vi "Available_Machines.vi"(1 "Row Number":i32) -> (0 "Machine Names":string[](array[string]))   [LabVIEW 2010]
uses:
  ADAM Controls/Channel_names.ctl
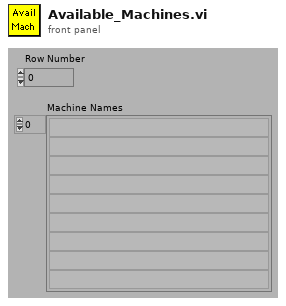
[diagram p1: front panel]
types:
  T1 = typedef "Channel_names.ctl" = enum16{"Active Only", "Active + Off", "All Channels"}
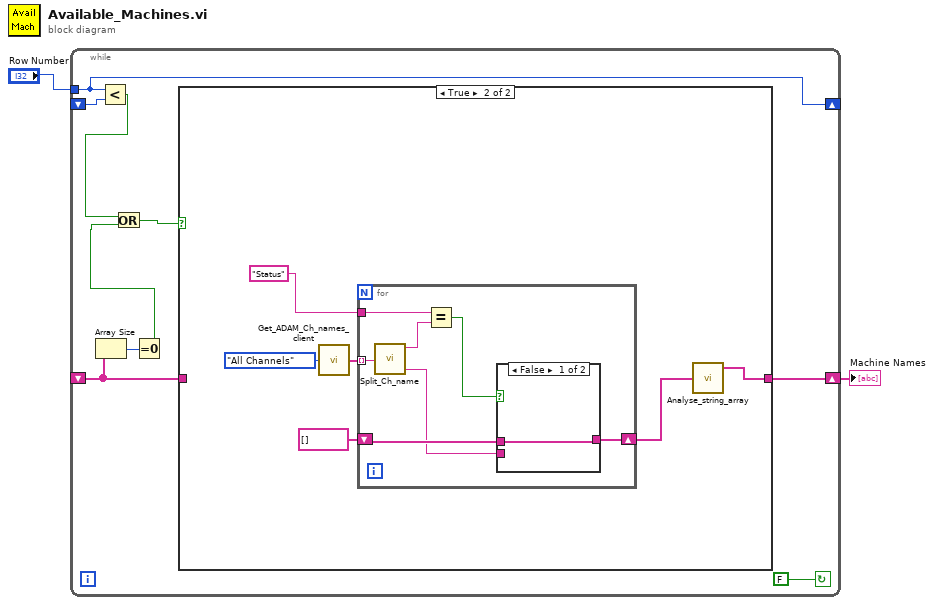
[diagram p0: block diagram]
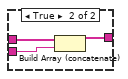
[diagram p3: hidden frame]
diagram:
  n1 = while {
    tunnel: "Row Number" -> [w10]
    shift-left: _ -> [w11]
    shift-right: [w10] -> _
    shift-left: _ -> [w4]
    shift-right: [w6] -> w1
    stop <- FALSE continue-if-true
    n2 = Array Size(array=w4) -> (size(s)=w9:i32)
    n3 = Less?(x=w10, y=w11) -> (x < y?=w7:bool)
    n4 = Equal To 0?(x=w9) -> (x = 0?=w8:bool)
    n5 = Or(x=w7, y=w8) -> (x .or. y?=w5:bool)
    n6 = case shown="True" w5 {
      tunnel: [w12 w14] -> w6
      tunnel: w4 -> [w12 _]
      frame False {
      }
      frame True {
        n7 = call "Get_ADAM_Ch_names_client.vi"("Channel names set"=Channel_names."All Channels") -> ("Ch names"=w17:string[])
        n8 = for {
          tunnel: w17 -> [w25] mode=indexing
          shift-right: [w21] -> w15
          shift-left: string[] [] -> [w22]
          tunnel: "Status" ("Substring") -> [w19]
          n9 = call "Split_Ch_name.vi"("Ch name"=w25) -> ("Top level"=w24:string, "Low level"=w20:string)  [unwired: 1 out]
          n10 = Equal?(x=w19, y=w24) -> (x = y?=w23:bool)
          n11 = case shown="False" w23 {
            tunnel: w22 -> [w26 w29]
            tunnel: [w26 w28] -> w21
            tunnel: w20 -> [_ w27]
            frame False {
            }
            frame True {
              n12 = Build Array (concatenate)(w29, w27) -> (w28:string[])
            }
          }
        }
        n13 = call "Analyse_string_array.vi"("String array"=w15) -> ("Unique strings"=w14:string[])  [unwired: 2 out]
      }
    }
  }
  "Machine Names" <- w1
